vi "MainVI_Reference_Action_SLM.vi"(0 "VI Ref IN":refnum<vi>, 2 "Action":u16(ring) items=["Read", "Initialize"]) -> (4 "VI Reference":refnum<vi>)   [LabVIEW 2014]
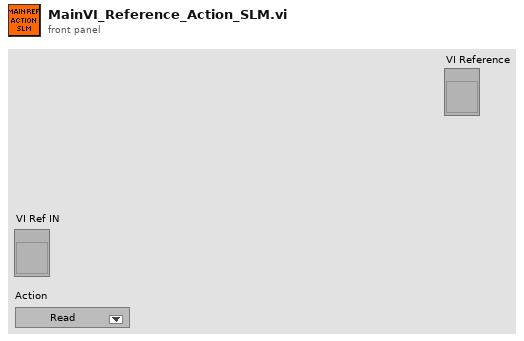
[diagram p1: front panel]
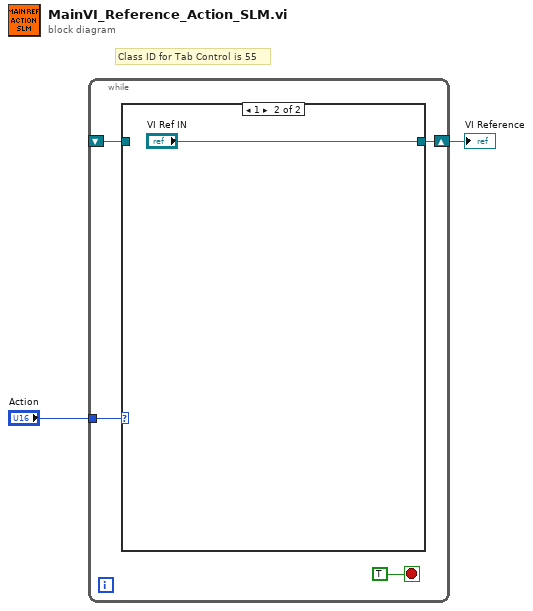
[diagram p0: block diagram]
diagram:
  # "Class ID for Tab Control is 55"
  n1 = while {
    tunnel: "Action" -> [w5]
    shift-right: [w4] -> w1
    shift-left: _ -> [w3]
    stop <- TRUE stop-if-true
    n2 = case shown="1" w5 {
      tunnel: [w7 "VI Ref IN"] -> w4
      tunnel: w3 -> [w7 _]
      frame 0, Default {
      }
      frame 1 {
      }
    }
  }
  "VI Reference" <- w1
